vi "Init DO DAQ v2.vi"(8 "error in":errorcluster, 10 "DAQChan[]":T1[](array[typedef])) -> (0 "error out":errorcluster, 3 "DO TaskRefs":refnum<k21>[](array[refnum]))   [LabVIEW 2017]
doc: "Developed by Kevin Thompson\nThompson Engineering, LLC\nkevin@thompsonengineering.net"
uses:
  Digital DAQChan--cluster.ctl
  <vilib>/DAQmx/create/channels.llb/DAQmx Create Channel (DO-Digital Output).vi
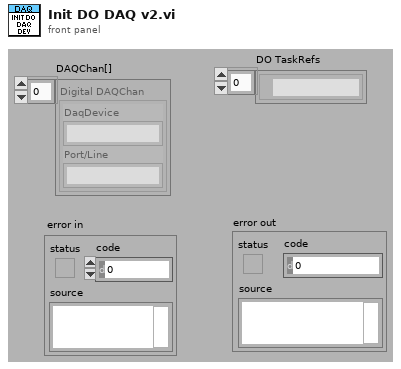
[diagram p1: front panel]
types:
  T1 = typedef "Digital DAQChan--cluster.ctl" = cluster{"DaqDevice":string, "Port/Line":string}
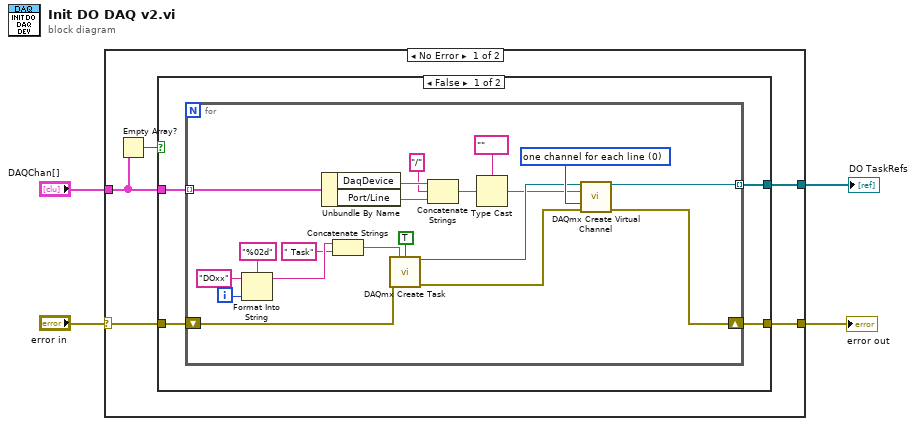
[diagram p0: block diagram]
diagram:
  n1 = case shown="No Error" "error in" {
    selector: "error in" -> [w7 w35]
    tunnel: "DAQChan[]" -> [w5 _]
    tunnel: [w9 w35] -> w3
    tunnel: [w8 _] -> w1
    frame No Error {
      n2 = Empty Array?(array=w5) -> (empty?=w6:bool)
      n3 = case shown="False" w6 {
        tunnel: w5 -> [w13 _]
        tunnel: [w12 w34] -> w9
        tunnel: [w11 _] -> w8
        tunnel: w7 -> [w10 w34]
        frame False {
          n4 = for {
            tunnel: w13 -> [w33] mode=indexing
            shift-right: [w14] -> w12
            shift-left: w10 -> [w20]
            tunnel: [w17] -> w11 mode=indexing
            i -> [w21]
            w19 = 0 items=["one channel for each line", "one channel for all lines"] ("line grouping")
            n5 = Format Into String(format string="%02d", initial string="DOxx", w21) -> (resulting string=w27:string)  [unwired: 1 in, 1 out]
            n6 = Unbundle By Name(w33) -> ("DaqDevice"=w32:string, "Port/Line"=w30:string)
            n7 = Concatenate Strings(w27, " Task" ("string")) -> (w26:string)
            n8 = call <vilib>:"DAQmx Create Task.vi"("new task name"=w26, "auto cleanup"=TRUE, "error in"=w20) -> ("task out"=w18:refnum<k21>, "error out"=w15:errorcluster)  [unwired: 11 in]
            n9 = Concatenate Strings(w32, "/", w30) -> (w28:string)
            n10 = Type Cast(type=tag "" ("PhysChan"), x=w28) -> (*(type *) &x=w16:tag)
            n11 = call-poly <vilib>:"DAQmx Create Virtual Channel.vi"("task in"=w18, "lines"=w16, "line grouping"=w19, "error in"=w15) -> ("task out"=w17:refnum<k21>, "error out"=w14:errorcluster)  [unwired: 10 in]
          }
        }
        frame True {
        }
      }
    }
    frame Error {
    }
  }
  "error out" <- w3
  "DO TaskRefs" <- w1
